vi "Set Main Settings.vi"(8 "error in (no error)":errorcluster, 10 "Main Settings":T1 {"Dummy Vrms" format="%.2g"}, 11 "Config in":refnum<class "Config.lvclass">) -> (0 "error out":errorcluster, 3 "Config out":refnum<class "Config.lvclass">)   [LabVIEW 2019, in "Config.lvclass"]
doc: "Developed by Kevin Thompson\nkevin@thompsonengineering.net\n\nCopyright 2018-2020\nThompson Engineering, LLC"
uses:
  Config.lvclass
  Main/DataTypes/Settings--cluster.ctl
  Main/support/Data Algorithms/subvis/DataTypes/Gain control.ctl
  Main/support/Data Algorithms/subvis/DataTypes/ESR scaling--cluster.ctl
  Config.lvclass/Config.ctl
  Main/Main.lvclass
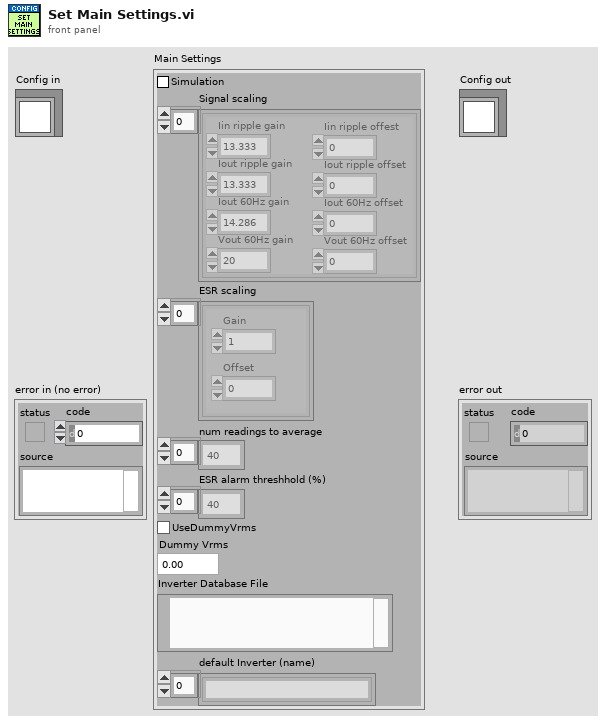
[diagram p1: front panel]
types:
  T1 = typedef "Main.lvclass/Settings--cluster.ctl" = cluster{"Simulation":bool, "Signal scaling":T2[], "ESR scaling":T3[], "num readings to average":i32[], "ESR alarm threshhold (%)":i32[], "UseDummyVrms":bool, "Dummy Vrms":dbl, "Inverter Database File":path, "default Inverter (name)":string[]}
  T2 = typedef "Main.lvclass/Gain control.ctl" = cluster{"Iin ripple gain":dbl, "Iout ripple gain":dbl, "Iout 60Hz gain ":dbl, "Vout 60Hz gain ":dbl, "Iin ripple offest":dbl, "Iout ripple offset":dbl, "Iout 60Hz offset":dbl, "Vout 60Hz offset":dbl}
  T3 = typedef "Main.lvclass/ESR scaling--cluster.ctl" = cluster{"Gain":dbl, "Offset":dbl}
  T4 = typedef "Config.lvclass/Config Settings.ctl" = cluster{"Application Settings":T5, "Main Settings":T1, "DAQ Settings":T6, "LogEngine Settings":T9}
  T5 = typedef "Application.lvclass/Settings--cluster.ctl" = cluster{"Simulation":bool}
  T6 = typedef "DAQ_Engine.lvclass/Settings--cluster.ctl" = cluster{"Simulation":bool, "Initial ErrReporting setting":i32, "Initial Measurement settings":T7, "Acquisition mode":T8, "DemoMode":bool}
  T7 = typedef "Measurement Config--cluster.ctl" = cluster{"Data Rate 9775":dbl, "Data Rate 9215":dbl, "Samples RMS 9215":u32, "Samples RMS 9775":u32}
  T8 = typedef "Acquisition Mode--cluster.ctl" = enum16{"3phase", "Single"}
  T9 = typedef "Log_Engine.lvclass/Settings--cluster.ctl" = cluster{"Simulation":bool, "TDMS_FolderPath":string, "CSV_FolderPath":string, "TDMS_FileName_Prefix":string, "CSV_FileName_Prefix":string, "TDMS_LogDuration(s)":dbl, "CSV_LogDuration(s)":dbl}[]
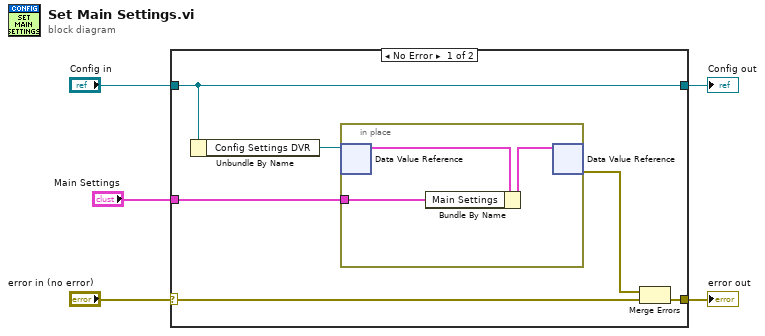
[diagram p0: block diagram]
diagram:
  n1 = case shown="No Error" "error in (no error)" {
    selector: "error in (no error)" -> [w7 w15]
    tunnel: [w6 w15] -> w1
    tunnel: [w9 w16] -> w4
    tunnel: "Config in" -> [w9 w16]
    tunnel: "Main Settings" -> [w8 _]
    frame No Error {
      n2 = Unbundle By Name(w9) -> ("Config Settings DVR"=w11:refnum<data-value>)
      n3 = in-place {
        in-place-border: w8 -> [w12]
        n4 = in-place-dvr #1(w11) -> (w14:T4)  [unwired: 1 out]
        n5 = Bundle By Name(cluster=w14, "Main Settings"=w12) -> (w13:T4)
        n6 = in-place-dvr #1(w13) -> (w10:errorcluster)  [unwired: 1 out]
      }
      n7 = Merge Errors(w10, w7) -> (w6:errorcluster)
    }
    frame Error {
    }
  }
  "error out" <- w1
  "Config out" <- w4
